vi "Part 1.vi"(11 "Input":string) -> (3 "Output":i64)   [LabVIEW 2021]
uses:
  <userlib>/_OpenG.lib/string/string.llb/Convert EOLs (String)__ogtk.vi
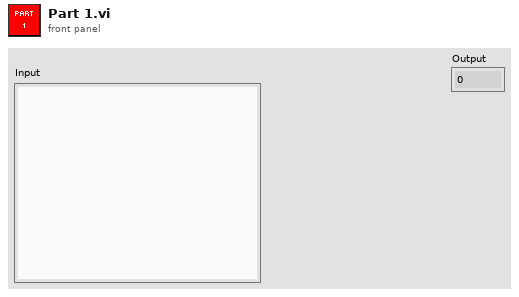
[diagram p1: front panel]
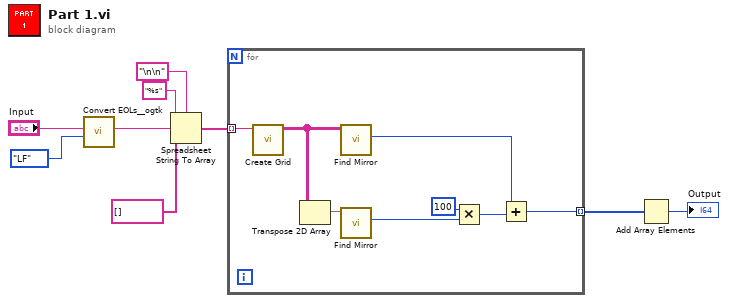
[diagram p0: block diagram]
diagram:
  n1 = call-poly <userlib>:"Convert EOLs__ogtk.vi"("Convert to:"=enum16{"CR", "LF", "CRLF"}."LF", "String in"="Input") -> ("String out"=w5:string)  [unwired: 9 in]
  n2 = Spreadsheet String To Array(delimiter (Tab)="\n\n", format string="%s", spreadsheet string=w5, array type (2D Dbl)=string[] []) -> (array=w3:string[])
  n3 = for {
    tunnel: w3 -> [w17] mode=indexing
    tunnel: [w15] -> w2 mode=indexing
    n4 = call "Create Grid.vi"("String"=w17) -> ("Array"=w16:string[][])  [unwired: 10 in]
    n5 = Transpose 2D Array(2D array=w16) -> (transposed array=w10:string[][])
    n6 = call "Find Mirror.vi"("Array in"=w16) -> ("element"=w14:i32)  [unwired: 8 in, 2 out]
    n7 = call "Find Mirror.vi"("Array in"=w10) -> ("element"=w12:i32)  [unwired: 8 in, 2 out]
    n8 = Multiply(x=100, y=w12) -> (x*y=w11:i32)
    n9 = Add(x=w14, y=w11) -> (x+y=w15:i32)
  }
  n10 = Add Array Elements(numeric array=w2) -> (sum=→"Output":i32)
